vi "test setting.vi"() -> ()   [LabVIEW 2013]
uses:
  lightfield-automation-labview/VIs/ClientServerMode/CS_LFAClassGlobal.vi
  lightfield-automation-labview/LightField Automation.lvclass
panel:
  out "Data":T1(array[cluster])
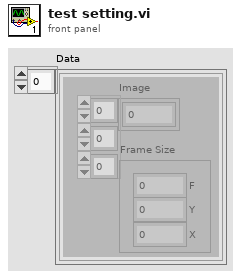
[diagram p1: front panel]
types:
  T1 = cluster{"Image":dbl[][][], "Frame Size":cluster{"F":i32, "Y":i32, "X":i32}}[]
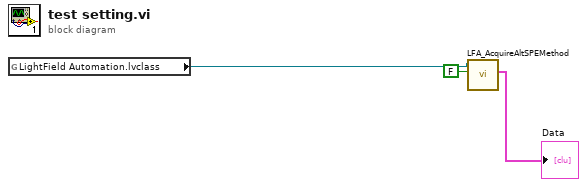
[diagram p0: block diagram]
diagram:
  n1 = global read "CS_LFAClassGlobal.vi" "LightField Automation.lvclass"() -> (w3:refnum<class "LightField Automation.lvclass">)
  n2 = call "LFA_AcquireAltSPEMethod.vi"("Delete File?"=FALSE, "LightField Automation in"=w3) -> ("Data"=→"Data":T1)  [unwired: 7 in, 2 out]
